vi "Arm Hardware.vi"(8 "error in (no error)":errorcluster, 9 "Request type":T1=enum."User command", 11 "Ni-Scope Digitizer in":refnum<class "Ni-Scope Digitizer.lvclass">) -> (0 "error out":errorcluster, 3 "Ni-Scope Digitizer out":refnum<class "Ni-Scope Digitizer.lvclass">)   [LabVIEW 2021, in "Ni-Scope Digitizer.lvclass"]
uses:
  Ni-Scope Digitizer.lvclass
  Ni-Scope Digitizer.lvclass/Ni-Scope Digitizer.ctl
  <instrlib>/niScope/Controls/niScope trigger source digital.ctl
  <instrlib>/niScope/Configure/Trigger/niScope Configure Trigger Digital.vi
  <instrlib>/niScope/Acquire/niScope Get Scaling Coefficients.vi
  <instrlib>/niScope/Configure/Trigger/niScope Configure Trigger Software.vi
  LabActor/Controllers/Process Controller/Request type.ctl
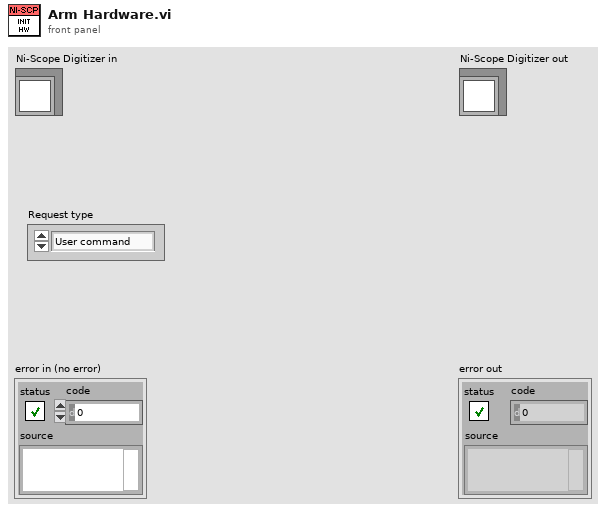
[diagram p1: front panel]
types:
  T1 = typedef "Request type.ctl" = enum16{"Process complete", "User command", "Auto-restart", "Error"}
  T2 = typedef "niScope trigger source digital.ctl" = string
  T3 = typedef "Pusle Driver Configuration.ctl" = cluster{"Post-trigger delay":dbl, "Post-trigger duration":dbl, "Rate":dbl, "Ranges":dbl[], "Re-name channels":string[], "Active channels":string, "External clock":bool}
  T4 = cluster{"offset":dbl, "gain":dbl, "reserved 1":dbl, "reserved 2":dbl}[]
  T5 = cluster{"offset":dbl, "gain":dbl, "reserved 1":dbl, "reserved 2":dbl}
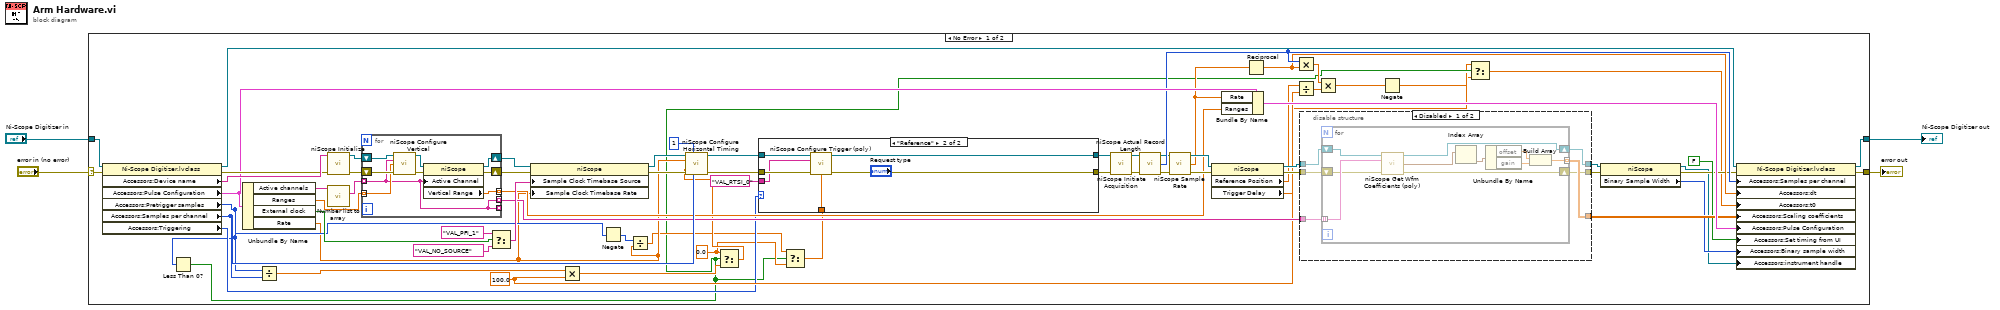
[diagram p0: block diagram]
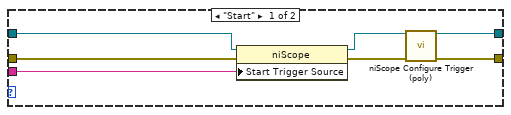
[diagram p2: hidden frame]
diagram:
  n1 = case shown="No Error" "error in (no error)" {
    selector: "error in (no error)" -> [w64 w114]
    tunnel: [w40 w114] -> w3
    tunnel: [w41 w113] -> w1
    tunnel: "Ni-Scope Digitizer in" -> [w46 w113]
    frame No Error {
      w14 = 0.0 ("t")
      w29 = 100.0 ("y")
      n2 = property class="Ni-Scope Digitizer.lvclass"(reference=w46, error in=w64) -> (reference out=w42:refnum<class "Ni-Scope Digitizer.lvclass">, error out=w65:errorcluster, "Accessors:Device name"=w66:string, "Accessors:Pulse Configuration"=w54:T3, "Accessors:Pretrigger samples"=w12:i32, "Accessors:Samples per channel"=w63:i32, "Accessors:Triggering"=w23:enum16{"Reference", "Start"})
      n3 = Less Than 0?(x=w12) -> (x < 0?=w8:bool)
      n4 = Unbundle By Name(w54) -> ("Active channels"=w69:string, "Ranges"=w67:dbl[], "External clock"=w58:bool, "Rate"=w10:dbl)
      n5 = Divide(x=w12, y=w63) -> (x/y=w17:dbl)
      n6 = call <instrlib>:"niScope Initialize.vi"("resource name"=w66, "error in"=w65) -> ("instrument handle"=w71:refnum<k15>, "error out"=w72:errorcluster)  [unwired: 2 in, 10 out]
      n7 = call "Number list to array.vi"("Number list"=w69) -> ("Full names"=w68:string[])  [unwired: 8 in, 2 out]
      n8 = for {
        tunnel: w67 -> [w110] mode=indexing
        shift-right: [w106] -> w61
        shift-left: w72 -> [w112]
        shift-right: [w108] -> w62
        shift-left: w71 -> [w111]
        tunnel: w68 -> [w104] mode=indexing
        tunnel: [w104] -> _ mode=indexing
        tunnel: [w105] -> w45 mode=indexing
        tunnel: [w104] -> w44 mode=indexing
        n9 = call <instrlib>:"niScope Configure Vertical.vi"("instrument handle"=w111, "channels"=w104, "vertical range"=w110, "error in"=w112) -> ("instrument handle out"=w109:refnum<k15>, "error out"=w107:errorcluster)  [unwired: 10 in]
        n10 = property class="niScope"(reference=w109, error in=w107, "Active Channel"=w104) -> (reference out=w108:refnum<k15>, error out=w106:errorcluster, "Vertical Range"=w105:dbl)
      }
      n11 = Select(t="VAL_PFI_1", s=w58, f="VAL_NO_SOURCE") -> (s? t:f=w55:string)
      n12 = property class="niScope"(reference=w62, error in=w61, "Sample Clock Timebase Source"=w55, "Sample Clock Timebase Rate"=w10) -> (reference out=w60:refnum<k15>, error out=w59:errorcluster)
      n13 = Multiply(x=w17, y=w29) -> (x*y=w16:dbl)
      n14 = Negate(x=w12) -> (-x=w11:i32)
      n15 = Divide(x=w11, y=w10) -> (x/y=w9:dbl)
      n16 = Select(t=w14, s=w8, f=w16) -> (s? t:f=w15:dbl)
      n17 = call <instrlib>:"niScope Configure Horizontal Timing.vi"("instrument handle"=w60, "number of records"=1, "min sample rate"=w10, "reference position"=w15, "error in"=w59, "min record length"=w63) -> ("instrument handle out"=w22:refnum<k15>, "error out"=w20:errorcluster)  [unwired: 1 in, 7 out]
      n18 = Select(t=w9, s=w8, f=w14) -> (s? t:f=w13:dbl)
      n19 = case shown="\"Reference\"" w23 {
        tunnel: w22 -> [w79 w85]
        tunnel: w20 -> [w74 w84]
        tunnel: T2 "VAL_RTSI_0" ("trigger source") -> [w73 w83]
        tunnel: [w78 w82] -> w19
        tunnel: [w77 w81] -> w18
        tunnel: w13 -> [_ w80]
        frame "Start" {
          n20 = property class="niScope"(reference=w79, error in=w74, "Start Trigger Source"=w73) -> (reference out=w76:refnum<k15>, error out=w75:errorcluster)
          n21 = call-poly <instrlib>:"niScope Configure Trigger (poly).vi"("instrument handle"=w76, "error in"=w75) -> ("instrument handle out"=w78:refnum<k15>, "error out"=w77:errorcluster)  [unwired: 12 in]
        }
        frame "Reference" {
          n22 = call-poly <instrlib>:"niScope Configure Trigger (poly).vi"("instrument handle"=w85, "trigger source"=w83, "error in"=w84, "trigger delay"=w80) -> ("instrument handle out"=w82:refnum<k15>, "error out"=w81:errorcluster)  [unwired: 10 in]
        }
      }
      n23 = call <instrlib>:"niScope Initiate Acquisition.vi"("instrument handle"=w19, "error in"=w18) -> ("instrument handle out"=w39:refnum<k15>, "error out"=w36:errorcluster)  [unwired: 12 in]
      n24 = call <instrlib>:"niScope Actual Record Length.vi"("instrument handle"=w39, "error in"=w36) -> ("instrument handle out"=w38:refnum<k15>, "actual record length"=w50:i32, "error out"=w37:errorcluster)  [unwired: 11 out]
      n25 = call <instrlib>:"niScope Sample Rate.vi"("instrument handle"=w38, "error in"=w37) -> ("instrument handle out"=w53:refnum<k15>, "actual sample rate"=w43:dbl, "error out"=w52:errorcluster)  [unwired: 11 out]
      n26 = property class="niScope"(reference=w53, error in=w52) -> (reference out=w35:refnum<k15>, error out=w34:errorcluster, "Reference Position"=w30:dbl, "Trigger Delay"=w7:dbl)
      n27 = Bundle By Name(cluster=w54, "Rate"=w43, "Ranges"=w45) -> (w51:T3)
      n28 = Reciprocal(x=w43) -> (1/x=w49:dbl)
      n29 = Multiply(x=w50, y=w49) -> (x*y=w48:dbl)
      n30 = Divide(x=w30, y=w29) -> (x/y=w31:dbl)
      n31 = disable-structure shown="Disabled" {
        disable-tunnel: w44 -> [w91 _]
        disable-tunnel: w35 -> [w90 w102]
        disable-tunnel: w34 -> [w89 w103]
        disable-tunnel: [w88 _] -> w33
        disable-tunnel: [w87 w102] -> w28
        disable-tunnel: [w86 w103] -> w27
        frame Disabled {
          n32 = for {
            tunnel: w91 -> [w93] mode=indexing
            shift-right: [w100] -> w86
            shift-left: w89 -> [w92]
            shift-right: [w101] -> w87
            shift-left: w90 -> [w94]
            tunnel: [w95] -> w88 mode=indexing
            n33 = call-poly <instrlib>:"niScope Get Wfm Coefficients (poly).vi"("instrument handle"=w94, "channels"=w93, "error in"=w92) -> ("instrument handle out"=w101:refnum<k15>, "coefficient info"=w99:T4, "error out"=w100:errorcluster)  [unwired: 10 in]
            n34 = Index Array(array=w99) -> (element=w98:T5)  [unwired: 1 in]
            n35 = Unbundle By Name(w98) -> ("offset"=w97:dbl, "gain"=w96:dbl)
            n36 = Build Array(w97, w96) -> (w95:dbl[])
          }
        }
        frame Enabled {
        }
      }
      n37 = Multiply(x=w48, y=w31) -> (x*y=w47:dbl)
      n38 = Negate(x=w47) -> (-x=w6:dbl)
      n39 = Select(t=w7, s=w8, f=w6) -> (s? t:f=w5:dbl)
      n40 = property class="niScope"(reference=w28, error in=w27) -> (reference out=w24:refnum<k15>, error out=w26:errorcluster, "Binary Sample Width"=w25:i32)
      n41 = property class="Ni-Scope Digitizer.lvclass"(reference=w42, error in=w26, "Accessors:Samples per channel"=w50, "Accessors:dt"=w49, "Accessors:t0"=w5, "Accessors:Scaling coefficients"=w33, "Accessors:Pulse Configuration"=w51, "Accessors:Set timing from UI"=FALSE ("Set timing from UI"), "Accessors:Binary sample width"=w25, "Accessors:instrument handle"=w24) -> (reference out=w41:refnum<class "Ni-Scope Digitizer.lvclass">, error out=w40:errorcluster)
    }
    frame Error {
    }
  }
  "error out" <- w3
  "Ni-Scope Digitizer out" <- w1
